vi "Close File.vi"(8 "error in (no error)":errorcluster, 11 "TDMS in":refnum<class "TDMS.lvclass">) -> (0 "error out":errorcluster, 3 "TDMS out":refnum<class "TDMS.lvclass">)   [LabVIEW 2020, in "TDMS.lvclass"]
uses:
  TDMS.lvclass
  TDMS.lvclass/TDMS.ctl
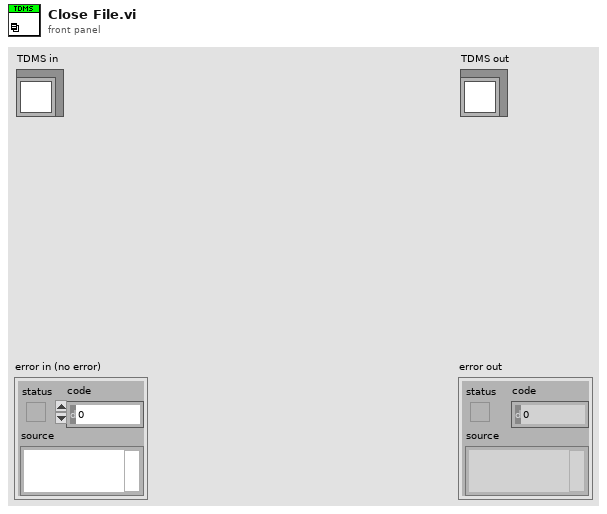
[diagram p1: front panel]
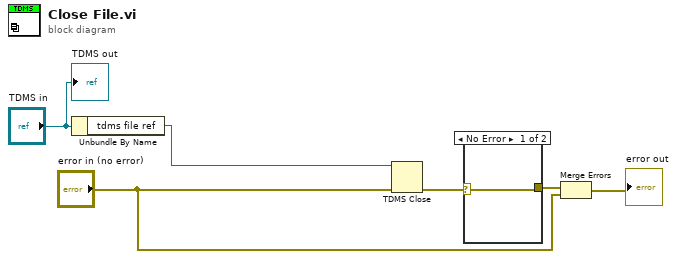
[diagram p0: block diagram]
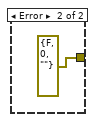
[diagram p2: hidden frame]
diagram:
  n1 = Unbundle By Name("TDMS in") -> ("tdms file ref"=w5:refnum<k34>)
  n2 = TDMS Close(8:"error in (no error)", 11:w5) -> (0:w4:errorcluster)  [unwired: 1 out]
  n3 = case shown="No Error" w4 {
    selector: w4 -> [w7 _]
    tunnel: [w7 errorcluster {"status"=FALSE, "code"=0, "source"=""} ("error in (no error)")] -> w3
    frame No Error {
    }
    frame Error {
    }
  }
  n4 = Merge Errors(w3, "error in (no error)") -> (→"error out":errorcluster)
  "TDMS out" <- "TDMS in"
